vi "client_main.vi"() -> ()   [LabVIEW 2020]
doc: "This vi writes TCP command from an already initialized TCP Connexion\nIf the write operation causes 56 or 66 code errors, reinitialize the TCP connexion and try to read data again . Number of maximal attempts is defined as input so that the state machine doesn't get stuck in an infinite loop"
panel:
  in  "IP":string
  in  "Port 2":u16
  in  "Port1":u16
  in  "stop":bool
  in  "Send button":bool
  out "Error OUT 2":errorcluster
  out "Respone":bool
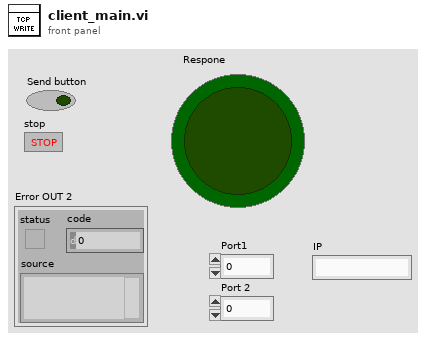
[diagram p1: front panel]
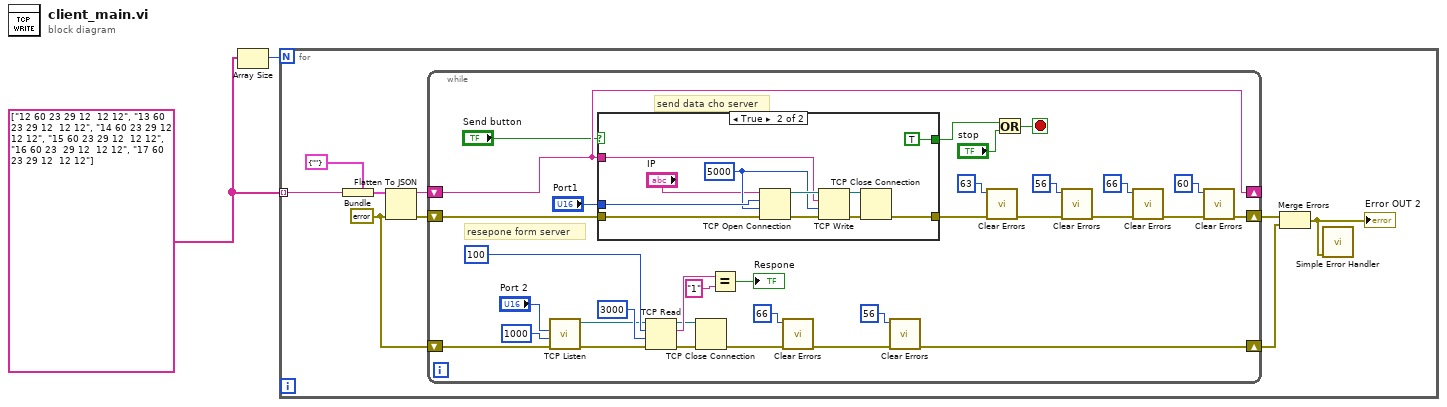
[diagram p0: block diagram]
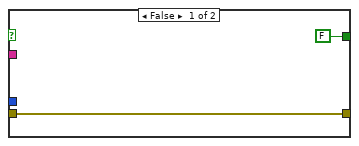
[diagram p2: hidden frame]
diagram:
  w1 = string[] ["12 60 23 29 12  12 12", "13 60 23 29 12  12 12", "14 60 23 29 12  12 12", "15 60 23 29 12  12 12", "16 60 23  29 12  12 12", "17 60 23 29 12  12 12"]
  n1 = Array Size(array=w1) -> (size(s)=w2:i32)
  n2 = for {
    N: w2 -> [_]
    tunnel: w1 -> [w7] mode=indexing
    w5 = errorcluster {"status"=FALSE, "code"=0, "source"=""} ("error out")
    n3 = Bundle(cluster=cluster{"Message":string} {"Message"=""}, "Message"=w7) -> (w8:cluster{"Message":string})
    n4 = Flatten To JSON(anything=w8, error in (no error)=w5) -> (JSON string=w6:string, 11:w4:errorcluster)  [unwired: 1 in]
    n5 = while {
      shift-right: [w33] -> _
      shift-left: w6 -> [w33]
      shift-right: [w40] -> w3
      shift-left: w5 -> [w41]
      shift-right: [w14] -> w11
      shift-left: w4 -> [w39]
      stop <- w22 stop-if-true
      # "resepone form server"
      # "send data cho server"
      n6 = call <vilib>:"TCP Listen.vi"("error in (no error)"=w41, "timeout ms (wait forever: -1)"=1000, "port"="Port 2") -> ("error out"=w29:errorcluster, "connection ID"=w28:refnum<k5>)  [unwired: 4 in, 3 out]
      n7 = case shown="True" "Send button" {
        tunnel: w33 -> [_ w53]
        tunnel: [w46 w49] -> w32
        tunnel: "Port1" -> [_ w52]
        tunnel: w39 -> [w46 w51]
        tunnel: [FALSE TRUE] -> w21
        frame False {
        }
        frame True {
          w50 = 5000 ("timeout ms (60000)")
          n8 = TCP Open Connection(address="IP", remote port or service name=w52, timeout ms (60000)=w50, error in (no error)=w51) -> (connection ID=w54:refnum<k5>, error out=w57:errorcluster)  [unwired: 1 in]
          n9 = TCP Write(connection ID=w54, data in=w53, error in (no error)=w57, 9:w50) -> (connection ID out=w55:refnum<k5>, error out=w56:errorcluster)  [unwired: 1 out]
          n10 = TCP Close Connection(connection ID=w55, error in (no error)=w56) -> (error out=w49:errorcluster)  [unwired: 1 in, 1 out]
        }
      }
      n11 = TCP Read(connection ID=w28, bytes to read=100, error in (no error)=w29, 9:3000 ("timeout ms (25000)")) -> (connection ID out=w26:refnum<k5>, data out=w43:string, error out=w27:errorcluster)  [unwired: 1 in]
      n12 = TCP Close Connection(connection ID=w26, error in (no error)=w27) -> (error out=w37:errorcluster)  [unwired: 1 in, 1 out]
      n13 = Equal?(x=w43, y="1") -> (x = y?=→"Respone":bool)
      n14 = call <vilib>:"Clear Errors.vi"("error in (no error)"=w37, "specific error code to clear (0: all)"=66) -> ("error out"=w36:errorcluster)  [unwired: 4 in, 1 out]
      n15 = call <vilib>:"Clear Errors.vi"("error in (no error)"=w36, "specific error code to clear (0: all)"=56) -> ("error out"=w40:errorcluster)  [unwired: 4 in, 1 out]
      n16 = call <vilib>:"Clear Errors.vi"("error in (no error)"=w32, "specific error code to clear (0: all)"=63) -> ("error out"=w20:errorcluster)  [unwired: 4 in, 1 out]
      n17 = Or(x=w21, y="stop") -> (x .or. y?=w22:bool)
      n18 = call <vilib>:"Clear Errors.vi"("error in (no error)"=w20, "specific error code to clear (0: all)"=56) -> ("error out"=w18:errorcluster)  [unwired: 4 in, 1 out]
      n19 = call <vilib>:"Clear Errors.vi"("error in (no error)"=w18, "specific error code to clear (0: all)"=66) -> ("error out"=w16:errorcluster)  [unwired: 4 in, 1 out]
      n20 = call <vilib>:"Clear Errors.vi"("error in (no error)"=w16, "specific error code to clear (0: all)"=60) -> ("error out"=w14:errorcluster)  [unwired: 4 in, 1 out]
    }
    n21 = Merge Errors(w11, w3) -> (w10:errorcluster)
    "Error OUT 2" <- w10
    n22 = call <vilib>:"Simple Error Handler.vi"("error in (no error)"=w10) -> ()  [unwired: 4 in, 5 out]
  }
